vi "DecodeMessage.vi"(5 "Message":string) -> (0 "Payload":string, 1 "Operation":u8, 2 "Device":u8)   [LabVIEW 2021]
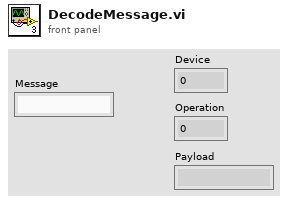
[diagram p1: front panel]
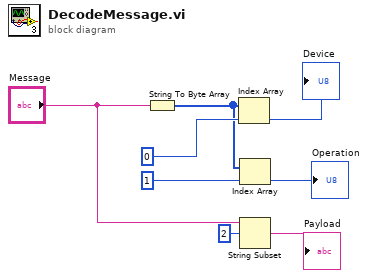
[diagram p0: block diagram]
diagram:
  n1 = String To Byte Array(string="Message") -> (unsigned byte array=w6:u8[])
  n2 = Index Array(array=w6, index=0) -> (element=→"Device":u8)
  n3 = Index Array(array=w6, index=1) -> (element=→"Operation":u8)
  n4 = String Subset(string="Message", offset (0)=2) -> (substring=→"Payload":string)  [unwired: 1 in]
